vi "network-find_mac_address.vi"(8 "error in (no error)":errorcluster, 10 "interface":string, 11 "ip_address":string) -> (0 "error out":errorcluster, 2 "mac_found?":bool, 3 "mac_address":string)   [LabVIEW 2015, in "lv-bin-windows.lvlib" / "v1.lvlib"]
uses:
  v1.lvlib
  <userlib>/antonio-alexander/lv-bin/lv-bin/public/api/v1/v1.lvlib
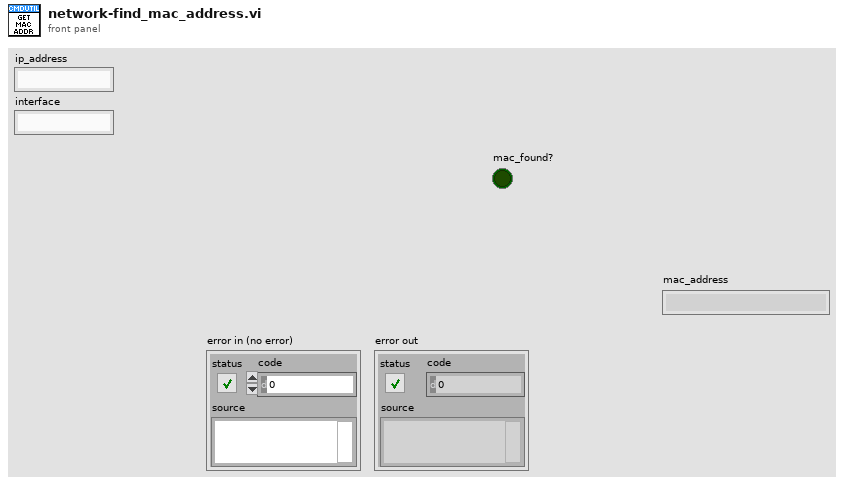
[diagram p1: front panel]
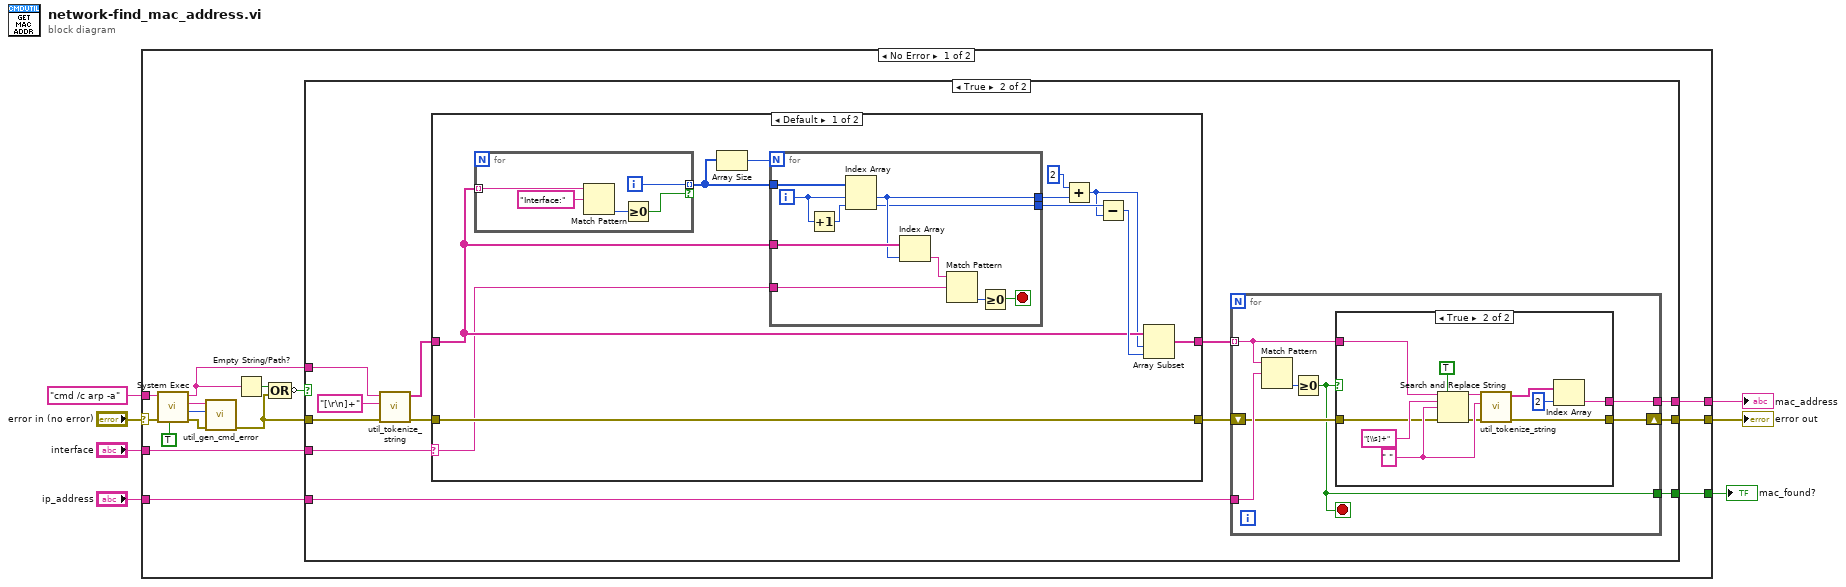
[diagram p0: block diagram]
diagram:
  n1 = case shown="No Error" "error in (no error)" {
    selector: "error in (no error)" -> [w16 w83]
    tunnel: "ip_address" -> [w17 _]
    tunnel: [w22 _] -> w5
    tunnel: [w21 _] -> w3
    tunnel: [w20 w83] -> w4
    tunnel: "cmd /c arp -a" ("format string") -> [w19 _]
    tunnel: "interface" -> [w18 _]
    frame No Error {
      n2 = call <vilib>:"System Exec.vi"("run minimized? (F)"=TRUE, "error in (no error)"=w16, "command line"=w19) -> ("error out"=w11:errorcluster, "return code"=w8:i32, "standard error"=w9:string, "standard output"=w14:string)  [unwired: 5 in]
      n3 = call <userlib>:"util_gen_cmd_error.vi"("error in (no error)"=w11, "return_code"=w8, "standard_error"=w9) -> ("error out"=w10:errorcluster)  [unwired: 8 in]
      n4 = Empty String/Path?(string/path=w14) -> (empty?=w13:bool)
      n5 = Compound Arithmetic op=OR(w13, w10) -> (invert w12:bool)
      n6 = case shown="True" w12 {
        tunnel: [_ w26] -> w22
        tunnel: [_ w27] -> w21
        tunnel: w14 -> [_ w30]
        tunnel: w17 -> [_ w24]
        tunnel: w10 -> [w23 w29]
        tunnel: [w23 w28] -> w20
        tunnel: w18 -> [_ w25]
        frame False {
        }
        frame True {
          n7 = call <userlib>:"util_tokenize_string.vi"("error in (no error)"=w29, "delimiter"="[\r\n]+" ("delimiter ([\\s\\t\\n\\r]+)"), "input_string"=w30) -> ("error out"=w35:errorcluster, "before_match []"=w32:string[])  [unwired: 6 in, 1 out]
          n8 = case shown="Default" w25 {
            selector: w25 -> [w36 _]
            tunnel: w35 -> [w37 w62]
            tunnel: w32 -> [w43 w63]
            tunnel: [w44 w63] -> w33
            tunnel: [w37 w62] -> w34
            frame Default {
              n9 = for {
                tunnel: w43 -> [w51] mode=indexing
                tunnel: [w48] -> w41 mode=indexing if=w47
                i -> [w48]
                n10 = Match Pattern(string=w51, regular expression="Interface:") -> (offset past match=w49:i32)  [unwired: 1 in, 3 out]
                n11 = Greater Or Equal To 0?(x=w49) -> (x >= 0?=w47:bool)
              }
              n12 = Array Size(array=w41) -> (size(s)=w40:i32)
              n13 = for {
                N: w40 -> [_]
                tunnel: w43 -> [w61]
                tunnel: w41 -> [w56]
                tunnel: w36 -> [w59]
                tunnel: [w55] -> w46
                tunnel: [w52] -> w42
                i -> [w54]
                stop <- w57 stop-if-true
                n14 = Increment(x=w54) -> (x+1=w53:i32)
                n15 = Index Array(array=w56, index #1=w54, index #2=w53) -> (element #1=w55:i32, element #2=w52:i32)
                n16 = Index Array(array=w61, index=w55) -> (element=w60:string)
                n17 = Match Pattern(string=w60, regular expression=w59) -> (offset past match=w58:i32)  [unwired: 1 in, 3 out]
                n18 = Greater Or Equal To 0?(x=w58) -> (x >= 0?=w57:bool)
              }
              n19 = Add(x=2, y=w46) -> (x+y=w39:i32)
              n20 = Subtract(x=w42, y=w39) -> (x-y=w45:i32)
              n21 = Array Subset(array=w43, index=w39, length=w45) -> (w44:string[])
            }
            frame "" {
            }
          }
          n22 = for {
            tunnel: w33 -> [w68] mode=indexing
            tunnel: w24 -> [w70]
            tunnel: [w67] -> w27
            tunnel: [w64] -> w26
            shift-right: [w65] -> w28
            shift-left: w34 -> [w66]
            stop <- w64 stop-if-true
            n23 = Match Pattern(string=w68, regular expression=w70) -> (offset past match=w69:i32)  [unwired: 1 in, 3 out]
            n24 = Greater Or Equal To 0?(x=w69) -> (x >= 0?=w64:bool)
            n25 = case shown="True" w64 {
              tunnel: w68 -> [_ w76]
              tunnel: [_ w75] -> w67
              tunnel: w66 -> [w71 w73]
              tunnel: [w71 w72] -> w65
              frame False {
              }
              frame True {
                w79 = " " ("replace string (\"\")")
                n26 = Search and Replace String(replace all?=TRUE ("replace all? (F)"), input string=w76, search string="[\\s]+", replace string=w79, error in=w73) -> (result string=w80:string, error out=w74:errorcluster)  [unwired: 3 in, 2 out]
                n27 = call <userlib>:"util_tokenize_string.vi"("error in (no error)"=w74, "delimiter"=w79, "input_string"=w80) -> ("error out"=w72:errorcluster, "before_match []"=w78:string[])  [unwired: 6 in, 1 out]
                n28 = Index Array(array=w78, index=2) -> (element=w75:string)
              }
            }
          }
        }
      }
    }
    frame Error {
    }
  }
  "error out" <- w4
  "mac_found?" <- w5
  "mac_address" <- w3
